vi "BOOLEAN_OPERATIONFRONT_PANLE.vi"() -> ()   [LabVIEW 2020]
panel:
  out "NOT":bool
  out "AND":bool
  out "OR":bool
  in  "INPUT":bool
  in  "INPUT":bool
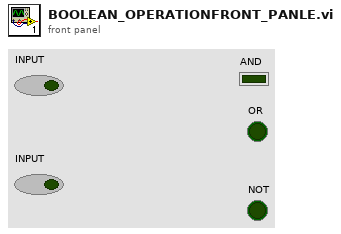
[diagram p1: front panel]
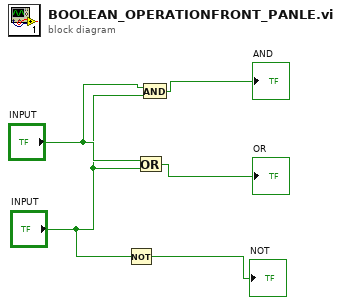
[diagram p0: block diagram]
diagram:
  n1 = Not(x="INPUT") -> (.not. x?=→"NOT":bool)
  n2 = Or(x="INPUT", y="INPUT") -> (x .or. y?=→"OR":bool)
  n3 = And(x="INPUT", y="INPUT") -> (x .and. y?=→"AND":bool)
